vi "XML.ListElementTextValues.vi"(8 "error in":errorcluster, 10 "element name":string, 11 "XML file path":path=path "C:/Projects/TM-OS/trunk/Design/XML_HW_config2.xml") -> (0 "error out":errorcluster, 2 "values":string[](array[string]))   [LabVIEW 2019, in "Tools.lvlib"]
uses:
  <vilib>/xml/Load XML File.vi
  <vilib>/xml/Close Reference(Node).vi
  Tools.lvlib
  <vilib>/xml/NI_XML.lvlib
  <resource>/objmgr/DOMUserDefRef.rc
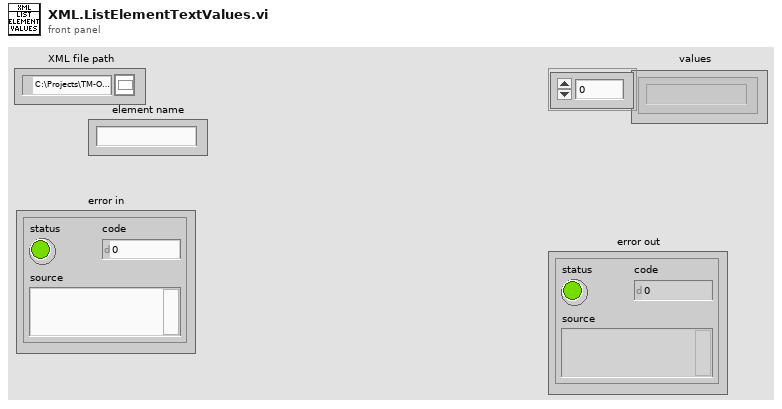
[diagram p1: front panel]
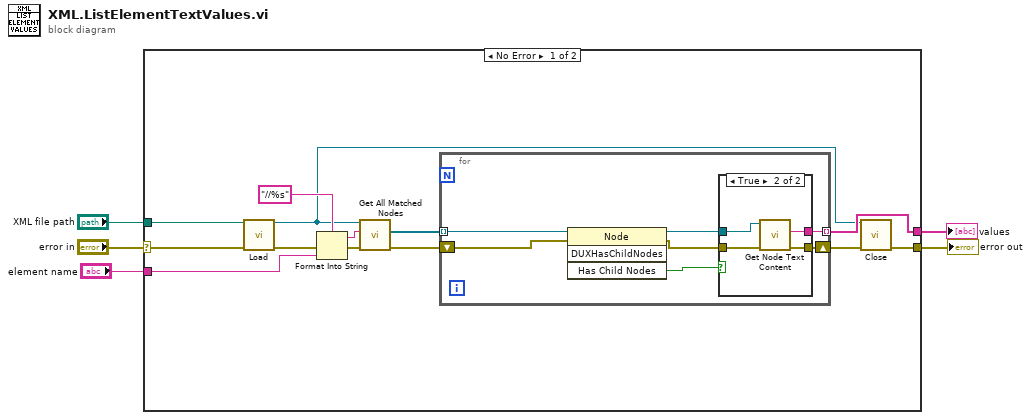
[diagram p0: block diagram]
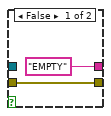
[diagram p2: hidden frame]
diagram:
  n1 = case shown="No Error" "error in" {
    selector: "error in" -> [w17 w32]
    tunnel: [w7 w32] -> w5
    tunnel: "XML file path" -> [w18 _]
    tunnel: [w9 _] -> w2
    tunnel: "element name" -> [w8 _]
    frame No Error {
      n2 = call-poly <vilib>:"Load.vi"("path to XML document"=w18, "error in (no error)"=w17) -> ("DOM document out"=w6:refnum<k20>, "error out"=w14:errorcluster)  [unwired: 11 in, 1 out]
      n3 = Format Into String(format string="//%s" ("XPath expression"), error in=w14, w8) -> (resulting string=w15:string, error out=w13:errorcluster)  [unwired: 1 in]
      n4 = call <vilib>:"Get All Matched Nodes.vi"("error in (no error)"=w13, "XPath expression"=w15, "node in"=w6) -> ("error out"=w10:errorcluster, "node result array"=w12:refnum<k20>[])  [unwired: 6 in, 1 out]
      n5 = for {
        tunnel: w12 -> [w20] mode=indexing
        tunnel: [w22] -> w9 mode=indexing
        shift-right: [w21] -> w11
        shift-left: w10 -> [w19]
        n6 = invoke class="Node" method="DUXHasChildNodes"(reference=w20, error in=w19) -> (reference out=w24:refnum<k20>, error out=w25:errorcluster, "Has Child Nodes"=w23:bool)  [unwired: 2 in, 1 out]
        n7 = case shown="True" w23 {
          tunnel: [w26 w31] -> w21
          tunnel: w25 -> [w26 w30]
          tunnel: w24 -> [_ w29]
          tunnel: ["EMPTY" w28] -> w22
          frame False {
          }
          frame True {
            n8 = call <vilib>:"Get Node Text Content.vi"("error in (no error)"=w30, "node in"=w29) -> ("error out"=w31:errorcluster, "node text"=w28:string)  [unwired: 7 in, 1 out]
          }
        }
      }
      n9 = call-poly <vilib>:"Close.vi"("error in (no error)"=w11, "node"=w6) -> ("error out"=w7:errorcluster)  [unwired: 7 in]
    }
    frame Error {
    }
  }
  "error out" <- w5
  "values" <- w2
